vi "Update Analysis Results.vi"(8 "error in (no error)":errorcluster, 10 "Results":variant, 11 "Hot And Cold Source Unit View in":refnum<class "Hot And Cold Source Unit View.lvclass">) -> (0 "error out":errorcluster, 3 "Hot And Cold Source Unit View out":refnum<class "Hot And Cold Source Unit View.lvclass">)   [LabVIEW 2013, in "Hot And Cold Source Unit View.lvlib" / "Hot And Cold Source Unit View.lvclass"]
uses:
  Hot And Cold Source Unit View.lvclass
  Hot And Cold Source Unit View.lvclass/Hot And Cold Source Unit View.ctl
  Common/Control Reference/Control Reference.lvlib
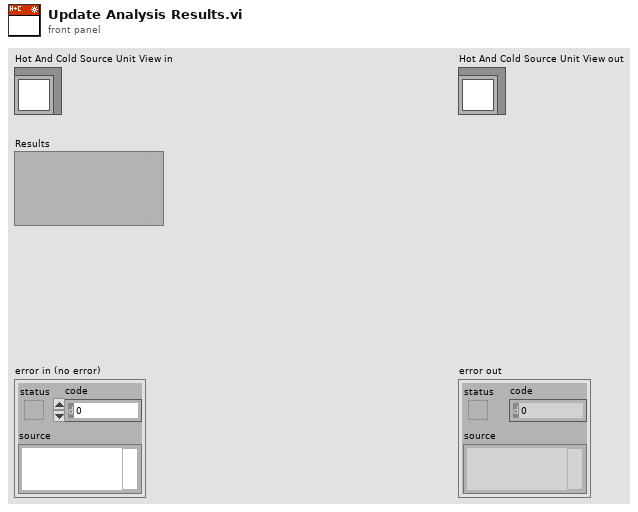
[diagram p1: front panel]
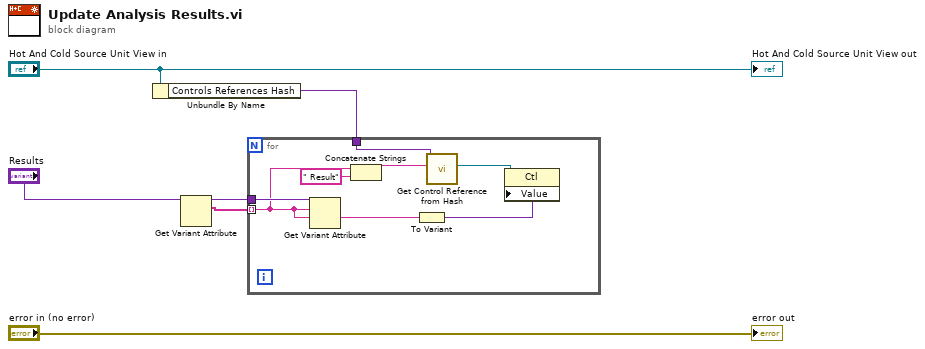
[diagram p0: block diagram]
diagram:
  n1 = Unbundle By Name("Hot And Cold Source Unit View in") -> ("Controls References Hash"=w2:variant)
  n2 = Get Variant Attribute(Variant="Results") -> (duplicate Variant=w4:variant, names=w3:string[])  [unwired: 3 in, 2 out]
  n3 = for {
    tunnel: w4 -> [w14]
    tunnel: w3 -> [w12] mode=indexing
    tunnel: w2 -> [w13]
    n4 = Get Variant Attribute(Variant=w14, name=w12, default value (empty Variant)=w12) -> (value=w8:string)  [unwired: 1 in, 3 out]
    n5 = Concatenate Strings(w12, " Result" ("string")) -> (w10:string)
    n6 = To Variant(anything=w8) -> (Variant=w7:variant)
    n7 = call "Get Control Reference from Hash.vi"("control label"=w10, "controls references hash"=w13) -> ("control reference"=w9:refnum<vi>)  [unwired: 6 in, 3 out]
    n8 = property class="Ctl"(reference=w9, "Value"=w7) -> ()  [unwired: 1 in, 2 out]
  }
  "error out" <- "error in (no error)"
  "Hot And Cold Source Unit View out" <- "Hot And Cold Source Unit View in"
